vi "Append to Text (subVI).vi"(7 "Error In":errorcluster, 9 "Text to append.":string, 10 "File Path Control":path) -> (0 "Error Out":errorcluster)   [LabVIEW 2013]
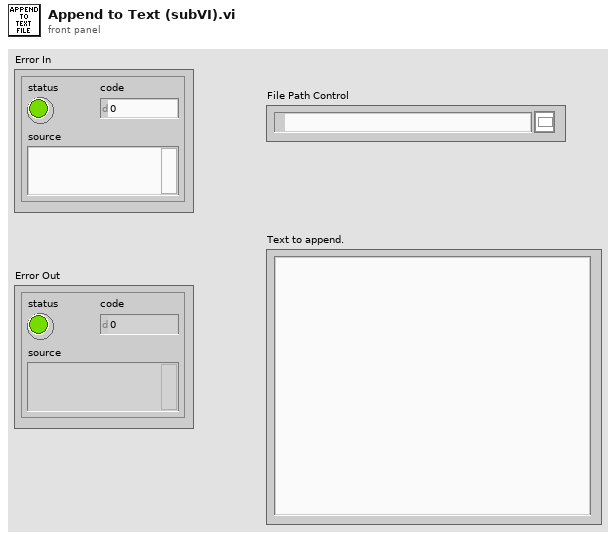
[diagram p1: front panel]
types:
  T1 = enum16{"open", "replace", "create", "open or create", "replace or create", "replace or create with confirmation"}
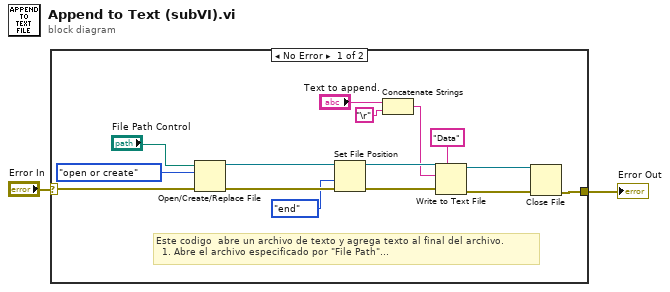
[diagram p0: block diagram]
diagram:
  n1 = case shown="No Error" "Error In" {
    selector: "Error In" -> [w17 w18]
    tunnel: [w3 w18] -> w1
    frame No Error {
      # "Este codigo  abre un archivo de texto y agrega texto al final del archivo.\n  1. Abre el archivo especificado por \"File Path\"..."
      n2 = Open/Create/Replace File(file path (use dialog)="File Path Control", error in=w17, operation (0:open)=T1."open or create") -> (refnum out=w13:refnum<file>, error out=w14:errorcluster)  [unwired: 3 in, 1 out]
      n3 = Set File Position(refnum=w13, from (0:start)=enum16{"start", "end", "current"}."end", error in=w14) -> (refnum out=w11:refnum<file>, error out=w10:errorcluster)  [unwired: 1 in]
      n4 = Concatenate Strings "Concatenate Strings"("Text to append.", "\r") -> (w6:string)
      n5 = Write to Text File(prompt (Choose or enter file path)="Data", file (use dialog)=w11, text=w6, error in=w10) -> (refnum out=w5:refnum<file>, error out=w4:errorcluster)  [unwired: 1 out]
      n6 = Close File(refnum=w5, error in=w4) -> (error out=w3:errorcluster)  [unwired: 1 out]
    }
    frame Error {
    }
  }
  "Error Out" <- w1
